vi "Data Source Simulator.vi"(8 "error in (no error)":errorcluster caption="Error In", 9 "Source":string, 10 "Identifiers In":map{string, T1}(c390), 11 "data":string[][](array[string])) -> (0 "error out":errorcluster caption="Error Out", 1 "Data":T2(c390), 2 "Identifiers Out":map{string, T1}(c390), 3 "Identifier List":T1[](array[typedef]), 5 "Identifiers":string)   [LabVIEW 2020]
uses:
  Global/Data Global/SDQ Data Type.ctl
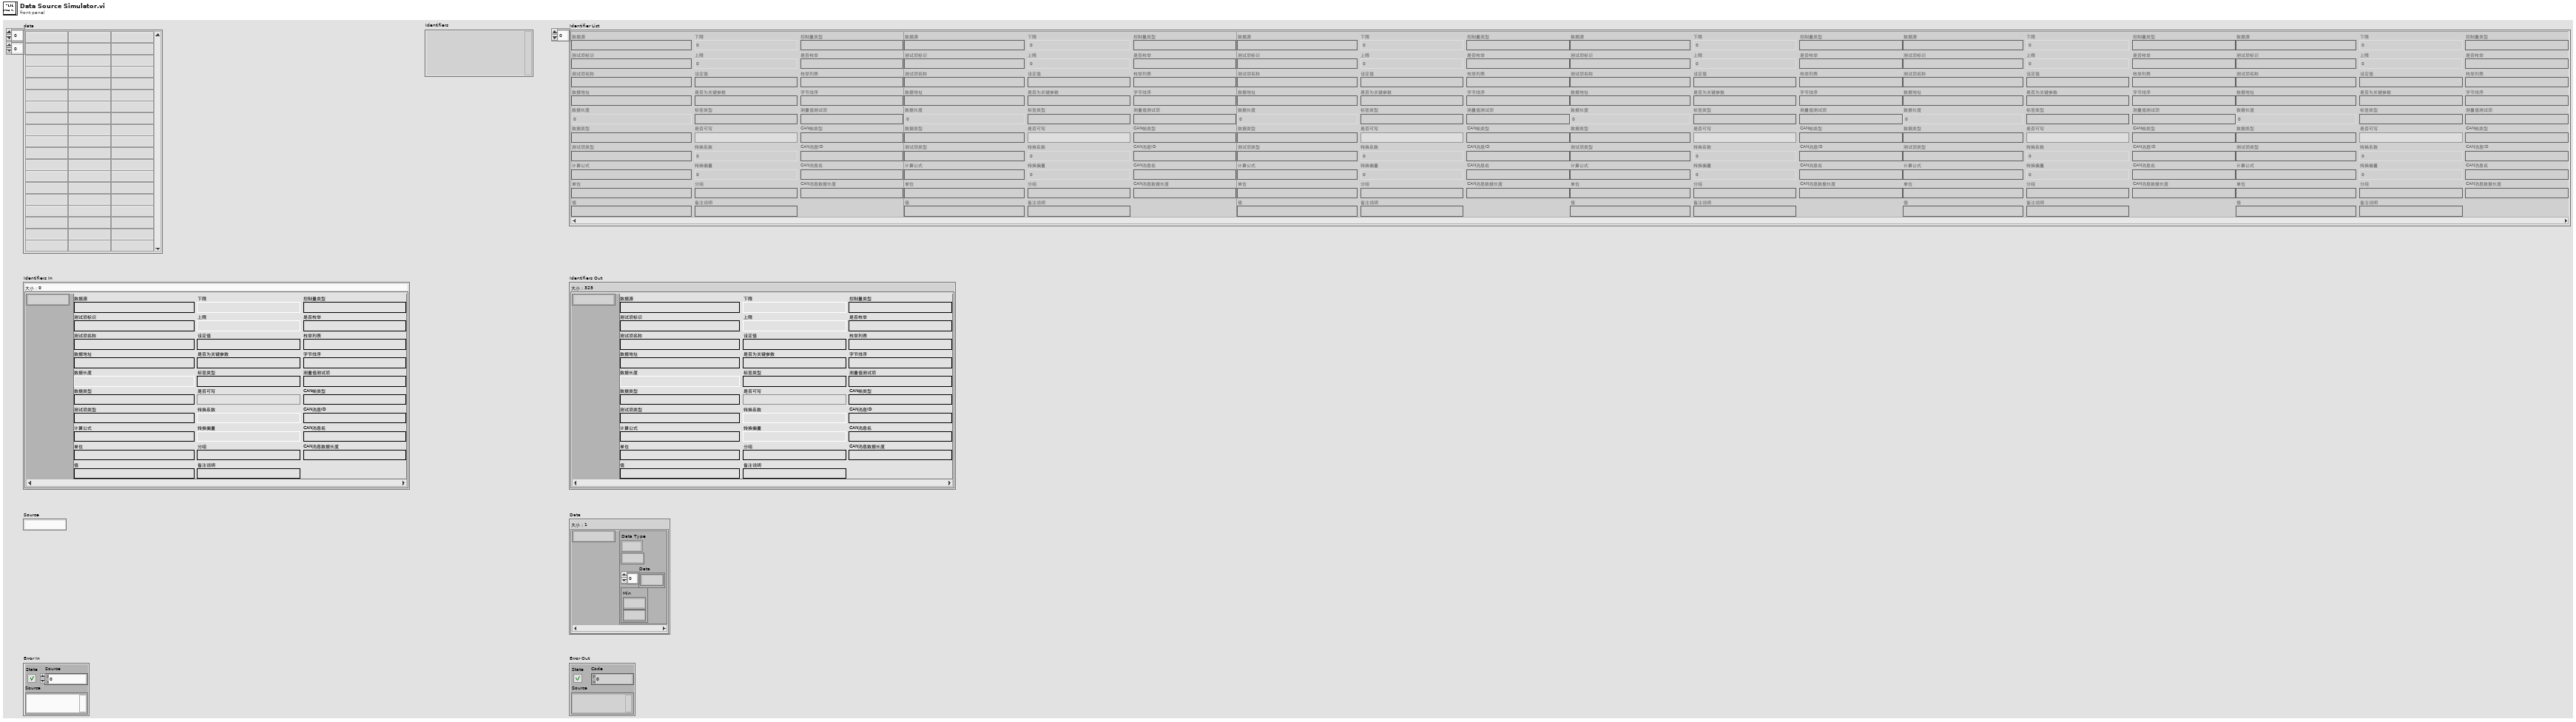
[diagram p1: front panel]
types:
  T1 = typedef "SDQ Data Type.ctl" = cluster{"CAN Length":string, "CAN Name":string, "CAN ID":string, "CAN Type":string, "Test Item":string, "Byte Order":string, "Instruction":string, "Control Type":string, "Group":string, "Offset":dbl, "Coefficient":dbl, "Write Enable":bool, "Lable Type":string, "Key?":string, "Set Value":string, "Upper":dbl, "Lower":dbl, "Unit":string, "Formula":string, "Test Item Type":string, "Length":i32, "Address":string, "Name":string, "Identifier":string, "Data Type":string, "Enumerate?":string, "Enumerate List":string, "Data":string, "Source":string}
  T2 = map{string, cluster{"Data Type":enum16{"I", "Q", "M", "D", "Count", "Timer"}, u16, "Data":u8[], cluster{"Min":u16, u16}}}
  T3 = cluster{"Data Type":enum16{"I", "Q", "M", "D", "Count", "Timer"}, "默认值 1":u16, "Data":u8[], cluster{"Min":i32, i32}}
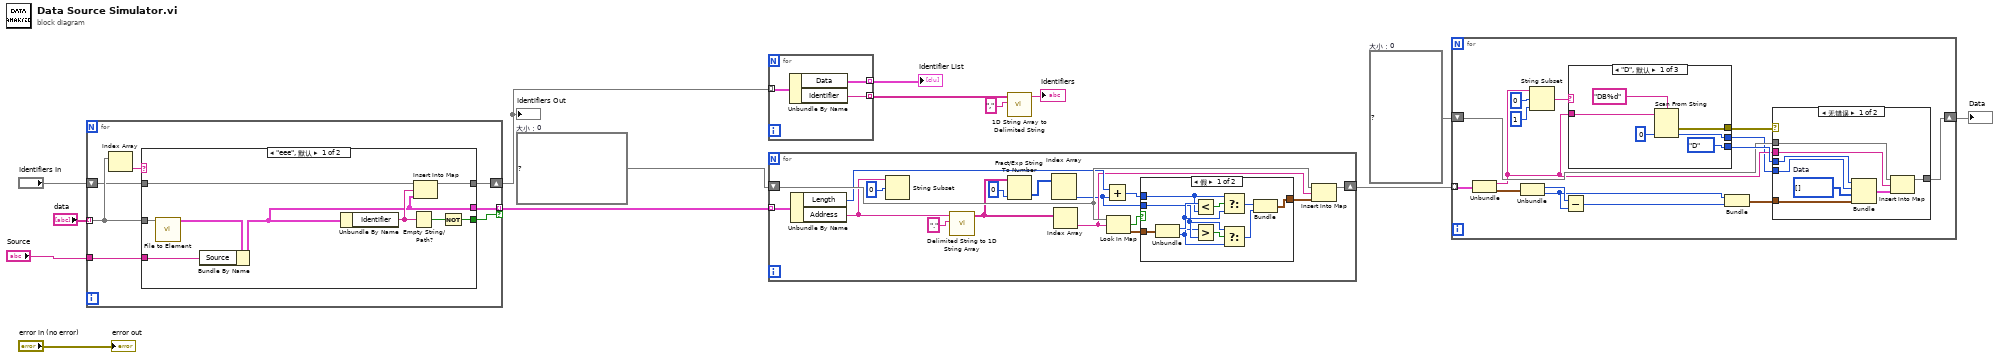
[diagram p0: block diagram]
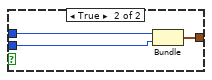
[diagram p2: hidden frame]
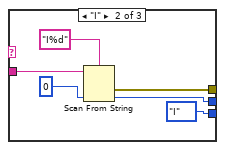
[diagram p4: hidden frame]
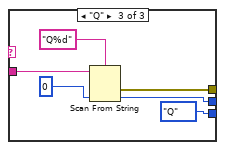
[diagram p5: hidden frame]
diagram:
  w9 = T2 {}  # 大小：0
  w11 = map{string, cluster{"Max":i32, "Min":i32}} {}  # 大小：0
  n1 = for {
    tunnel: "data" -> [w19] mode=indexing
    tunnel: [w21] -> w7 mode=indexing if=w20
    shift-right: [w16] -> w6
    shift-left: "Identifiers In" -> [w17]
    tunnel: "Source" -> [w15]
    n2 = Index Array(array=w19) -> (element=w18:string)  [unwired: 1 in]
    n3 = case shown="\"eee\", 默认" w18 {
      tunnel: w19 -> [w30 _]
      tunnel: [w23 _] -> w21
      tunnel: [w28 _] -> w20
      tunnel: w17 -> [w27 w31]
      tunnel: [w26 w31] -> w16
      tunnel: w15 -> [w22 _]
      frame "eee", Default {
        n4 = call "File to Element.vi"("Data In"=w30) -> ("Element Out"=w25:T1)  [unwired: 9 in, 1 out]
        n5 = Bundle By Name(cluster=w25, "Source"=w22) -> (w23:T1)
        n6 = Unbundle By Name(w23) -> ("Identifier"=w24:string)
        n7 = Empty String/Path?(string/path=w24) -> (empty?=w29:bool)
        n8 = Insert Into Map(map in=w27, key=w24, value=w23) -> (map out=w26:map{string, T1})  [unwired: 2 out]
        n9 = Not(x=w29) -> (.not. x?=w28:bool)
      }
      frame "" {
      }
    }
  }
  "Identifiers Out" <- w6
  n10 = for {
    tunnel: w6 -> [w34] mode=indexing
    tunnel: [w33] -> w5 mode=indexing
    tunnel: [w32] -> w4 mode=indexing
    n11 = Unbundle By Name(w34) -> ("Data"=w33:T1, "Identifier"=w32:string)
  }
  "Identifier List" <- w5
  n12 = for {
    tunnel: w7 -> [w50] mode=indexing
    shift-right: [w47] -> w10
    shift-left: w11 -> [w49]
    n13 = Unbundle By Name(w50) -> ("Length"=w48:i32, "Address"=w46:string)
    n14 = String Subset(string=w46, offset (0)=0 ("偏移量(0)")) -> ()  [unwired: 1 in, 1 out]
    n15 = call <vilib>:"Delimited String to 1D String Array.vi"("delimiter"=".", "delimited string"=w46) -> ("string array"=w37:string[])  [unwired: 9 in]
    n16 = Fract/Exp String To Number(string=w37, default (0 dbl)=0 ("默认(0 DBL)")) -> (number=w39:i32[])  [unwired: 2 in, 1 out]
    n17 = Index Array(array=w39) -> (element #2=w35:i32)  [unwired: 2 in, 1 out]
    n18 = Index Array(array=w37) -> (element=w36:string)  [unwired: 1 in]
    n19 = Add(x=w48, y=w35) -> (x+y=w38:i32)
    n20 = Look In Map(map=w49, key=w36) -> (key not found?=w44:bool, value=w43:cluster{"Max":i32, "Min":i32})  [unwired: 1 in]
    n21 = case shown="假" w44 {
      tunnel: w43 -> [w60 _]
      tunnel: [w51 w61] -> w42
      tunnel: w38 -> [w56 w63]
      tunnel: w35 -> [w55 w62]
      frame False {
        n22 = Unbundle(w60) -> ("Max"=w58:i32, "Min"=w54:i32)
        n23 = Less?(x=w58, y=w56) -> (x < y?=w59:bool)
        n24 = Greater?(x=w54, y=w55) -> (0:w57:bool)
        n25 = Select(t=w56, s=w59, f=w58) -> (s? t:f=w53:i32)
        n26 = Select(t=w55, s=w57, f=w54) -> (s? t:f=w52:i32)
        n27 = Bundle("Max"=w53, "Min"=w52) -> (w51:cluster{"Max":i32, "Min":i32})  [unwired: 1 in]
      }
      frame True {
        n28 = Bundle(w63, "String"=w62) -> (w61:cluster{i32, "String":i32})  [unwired: 1 in]
      }
    }
    n29 = Insert Into Map(map in=w49, key=w36, value=w42) -> (map out=w47:map{string, cluster{"Max":i32, "Min":i32}})  [unwired: 2 out]
  }
  n30 = call <vilib>:"1D String Array to Delimited String.vi"("delimiter"=",", "string array"=w4) -> ("delimited string"=→"Identifiers":string)  [unwired: 9 in]
  n31 = for {
    tunnel: w10 -> [w74] mode=indexing
    shift-right: [w67] -> w8
    shift-left: w9 -> [w68]
    n32 = Unbundle(w74) -> ("Data Type"=w66:string, w73:cluster{"Max":i32, "Min":i32})
    n33 = Unbundle(w73) -> ("Max"=w72:i32, "Min"=w71:i32)
    n34 = String Subset(string=w66, offset (0)=0 ("偏移量(0)"), length (rest)=1 ("长度（剩余）")) -> (substring=w76:string)
    n35 = Subtract(x=w72, y=w71) -> (x-y=w70:i32)
    n36 = case shown="\"D\", 默认" w76 {
      tunnel: [enum16{"I", "Q", "M", "D", "Count", "Timer"}."D" ("Data Type") enum16{"I", "Q", "M", "D", "Count", "Timer"}."I" ("Data Type") enum16{"I", "Q", "M", "D", "Count", "Timer"}."Q" ("Data Type")] -> w75
      tunnel: w66 -> [w91 w96 w102]
      tunnel: [w89 w95 w101] -> w65
      tunnel: [w88 w94 w100] -> w64
      frame "D", Default {
        n37 = Scan From String(format string="DB%d" ("格式字符串"), input string=w91, default 1=u16 0 ("默认值 1")) -> (error out=w88:errorcluster, output 1=w89:u16)  [unwired: 2 in, 2 out]
      }
      frame "I" {
        n38 = Scan From String(format string="I%d" ("格式字符串"), input string=w96, default 1=u16 0 ("默认值 1")) -> (error out=w94:errorcluster, output 1=w95:u16)  [unwired: 2 in, 2 out]
      }
      frame "Q" {
        n39 = Scan From String(format string="Q%d" ("格式字符串"), input string=w102, default 1=u16 0 ("默认值 1")) -> (error out=w100:errorcluster, output 1=w101:u16)  [unwired: 2 in, 2 out]
      }
    }
    n40 = Bundle("Min"=w71, w70) -> (w69:cluster{"Min":i32, i32})  [unwired: 1 in]
    n41 = case shown="无错误" w64 {
      tunnel: w75 -> [w86 _]
      tunnel: w69 -> [w84 _]
      tunnel: w68 -> [w83 w87]
      tunnel: [w82 w87] -> w67
      tunnel: w66 -> [w80 _]
      tunnel: w65 -> [w79 _]
      frame No Error {
        w85 = u8[] []  # Data
        n42 = Bundle("Data Type"=w86, "默认值 1"=w79, "Data"=w85, w84) -> (w81:T3)  [unwired: 1 in]
        n43 = Insert Into Map(map in=w83, key=w80, value=w81) -> (map out=w82:T2)  [unwired: 2 out]
      }
      frame Error {
      }
    }
  }
  "Data" <- w8
  "error out" <- "error in (no error)"
